vi "CommonCmds.vi"(0 "VISA IN":refnum<visa-resource-name>="PNA", 5 "error in":errorcluster, 7 "Cmds":string(combo)="SYST:ERR?") -> (14 "VISA Out":refnum<visa-resource-name>, 16 "Response":string, 19 "error out":errorcluster={"status"=TRUE, "code"=-1073807346, "source"="VISA Write in CommonCmds.vi"})   [LabVIEW 2018, in "PNA-X.lvlib"]
uses:
  PNA-X.lvlib
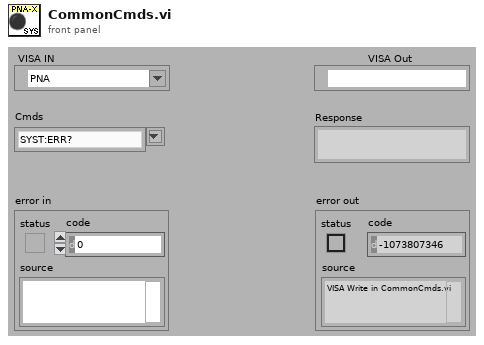
[diagram p1: front panel]
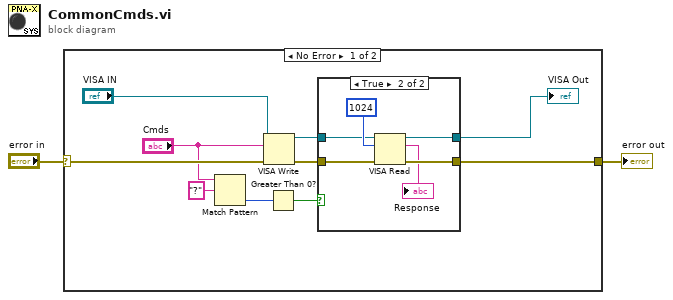
[diagram p0: block diagram]
diagram:
  n1 = case shown="No Error" "error in" {
    selector: "error in" -> [w7 w21]
    tunnel: [w8 w21] -> w1
    frame No Error {
      n2 = Match Pattern(string="Cmds", regular expression="?") -> (offset past match=w4:i32)  [unwired: 1 in, 3 out]
      n3 = VISA Write(VISA resource name="VISA IN", write buffer="Cmds", error in (no error)=w7) -> (VISA resource name out=w10:refnum<visa-resource-name>, error out=w11:errorcluster)  [unwired: 1 out]
      n4 = Greater Than 0?(x=w4) -> (x > 0?=w5:bool)
      n5 = case shown="True" w5 {
        tunnel: w11 -> [w14 w20]
        tunnel: w10 -> [w13 w18]
        tunnel: [w13 w17] -> w9
        tunnel: [w14 w16] -> w8
        frame False {
        }
        frame True {
          n6 = VISA Read(VISA resource name=w18, byte count=1024, error in (no error)=w20) -> (VISA resource name out=w17:refnum<visa-resource-name>, read buffer=→"Response":string, error out=w16:errorcluster)  [unwired: 1 out]
        }
      }
      "VISA Out" <- w9
    }
    frame Error {
    }
  }
  "error out" <- w1
